vi "Form_motor_command.vi"(9 "Command selection":u16(ring)=1 items=["Move", "Get Motor Completed Steps (Q[0..3]C)", "Get Motor Direction (Q[0..3]D)", "Get Motor Step Rate: (Q[0..3]R)", "Get Switch State: (Q[0..3]S)"], 10 "Move parameters":T1={"MOTOR NUMBER"=0, "Direction"=TRUE, "NUMBER OF  STEPS"=8000, "SPEED STEPS/SEC"=2000, "ACC/DECEL STEPS/SEC^2"=1000, "Move mode"=1, "EN/DIS?"=TRUE, "delay before \nread (ms)"=750, "Timeout before \nstop (ms)"=15000, "visa resource name"=""} {"Move mode" items=["Relative steps ##", "Search switch"]; "ACC/DECEL STEPS/SEC^2" max=4000; "SPEED STEPS/SEC" min=20 max=4000 step=10; "MOTOR NUMBER" max=3 step=1}) -> (3 "Motor Command Formed":string)   [LabVIEW 2020]
panel:
  in  "Commands strings":string[](array[string])=["M01-R1000:100:1000\n", "Q0C", "Q0D", "Q0S", "Q0D"]
  # "Emergency Stop:\n *      [M]|Motor # [0-3]|Motor State [0]|[EOT]\n *\n *  Get Motor Completed Steps:\n *      [Q]|Motor # [0-3]|[C]|[EOT]\n *  Get Motor Direction:\n *      [Q]|Motor # [0-3]|[D]|[EOT]\n *  Get Motor Step Rate:\n *      [Q]|Motor # [0-3]|[R]|[EOT]\n *  Get Switch State:\n *      [Q]|Motor # [0-3]|[S]|[EOT]\n *\n *  Set Emergency Ramp Multiplier:\n *      [V]|Motor # [0-3]|[E]|Multiplier [uint]|[EOT]\n *\n *  Reset the arduino:\n *      [R]|[EOT]\n *"
  # "*  Move:\n *      [M]|Motor # [0-3]|Motor State [1]|Motor Direction [+,-]|Type of Move [R,S]|# Steps [uint]|Delimiter [:]|Max. Rate [uint]|Delimiter [:]|Ramp Slope [uint]|Delimiter [:] (optional)|# Positions [uint] (optional)|[EOT]\n *          * type of move: R --> relative move, S --> switch move\n *          * if number of steps is 0 --> free run\n *          * if Ramp Slope == 0 -> no ramp (start at max. rate)\n *          * may specify the number of position to move for a switch move.  if not specified, defaults to 1 position.\n *\n *  Emergency Stop:\n *      [M]|Motor # [0-3]|Motor State [0]|[EOT]\n *\n *  Get Motor Completed Steps:\n *      [Q]|Motor # [0-3]|[C]|[EOT]\n *  Get Motor Direction:\n *      [Q]|Motor # [0-3]|[D]|[EOT]\n *  Get Motor Step Rate:\n *      [Q]|Motor # [0-3]|[R]|[EOT]\n *  Get Switch State:\n *      [Q]|Motor # [0-3]|[S]|[EOT]\n *\n *  Set Emergency Ramp Multiplier:\n *      [V]|Motor # [0-3]|[E]|Multiplier [uint]|[EOT]\n */"
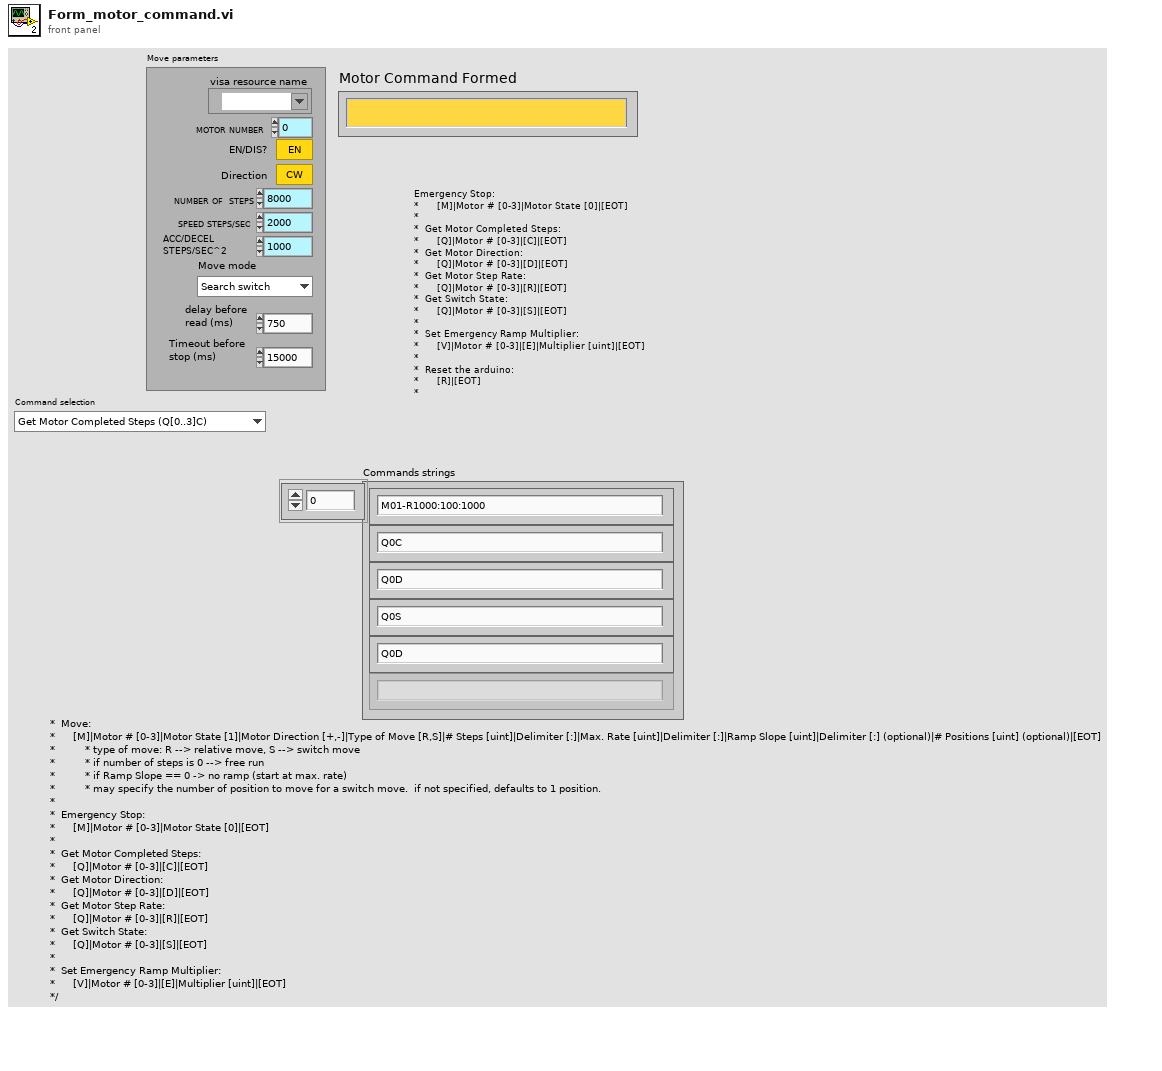
[diagram p1: front panel]
types:
  T1 = cluster{"MOTOR NUMBER":u8, "Direction":bool, "NUMBER OF  STEPS":u32, "SPEED STEPS/SEC":u16, "ACC/DECEL STEPS/SEC^2":u16, "Move mode":u16, "EN/DIS?":bool, "delay before \nread (ms)":u32, "Timeout before \nstop (ms)":u32, "visa resource name":refnum<visa-resource-name>}
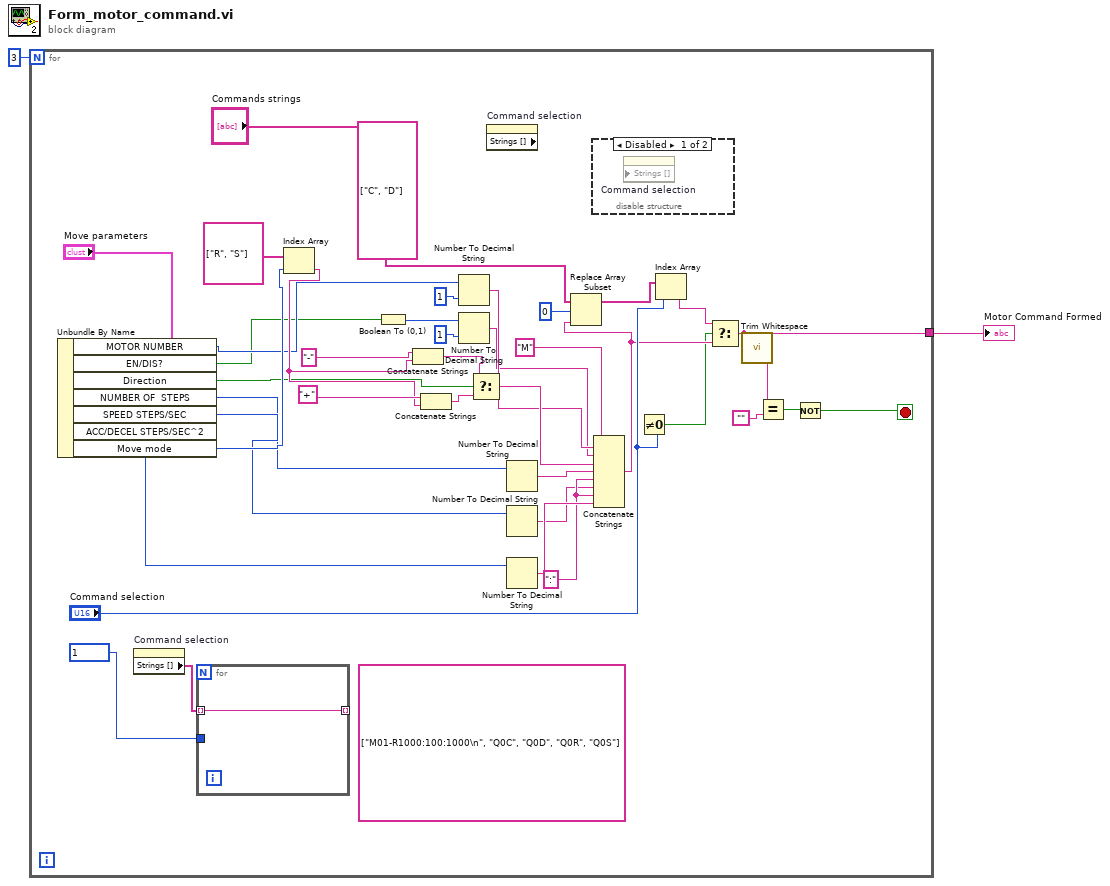
[diagram p0: block diagram]
diagram:
  n1 = for {
    N: 3 -> [_]
    tunnel: [w4] -> w1
    stop <- w5 stop-if-true
    (unwired) string[] ["M01-R1000:100:1000\n", "Q0C", "Q0D", "Q0R", "Q0S"] ("Commands strings")
    (unwired) string[] ["C", "D"]
    w22 = ":"
    n2 = Unbundle By Name("Move parameters") -> ("MOTOR NUMBER"=w14:u8, "EN/DIS?"=w12:bool, "Direction"=w30:bool, "NUMBER OF  STEPS"=w31:u32, "SPEED STEPS/SEC"=w32:u16, "ACC/DECEL STEPS/SEC^2"=w33:u16, "Move mode"=w41:u16)
    n3 = property on="Command selection" class="Ring (strict)"() -> ("Strings []"=w9:string[])  [unwired: 2 in, 2 out]
    n4 = for {
      tunnel: u16 1 ("Command selection") -> [_]
      tunnel: [w42] -> _ mode=indexing
      tunnel: w9 -> [w42] mode=indexing
    }
    n5 = Index Array(array=string[] ["R", "S"], index=w41) -> (element=w38:string)
    n6 = Boolean To (0,1)(Boolean=w12) -> (0, 1=w13:i16)
    n7 = Concatenate Strings("-", w38) -> (w35:string)
    n8 = Concatenate Strings("+", w38) -> (w40:string)
    n9 = Number To Decimal String(number=w14, width (-)=i16 1) -> (decimal integer string=w18:string)
    n10 = Number To Decimal String(number=w13, width (-)=i16 1) -> (decimal integer string=w11:string)
    n11 = Select(t=w35, s=w30, f=w40) -> (s? t:f=w27:string)
    n12 = property on="Command selection" class="Ring (strict)" props=["Strings []"]() -> ()  [unwired: 2 in, 3 out]
    n13 = Number To Decimal String(number=w31) -> (decimal integer string=w20:string)  [unwired: 1 in]
    n14 = Number To Decimal String(number=w32) -> (decimal integer string=w21:string)  [unwired: 1 in]
    n15 = Number To Decimal String(number=w33) -> (decimal integer string=w23:string)  [unwired: 1 in]
    n16 = disable-structure shown="Disabled" {
      frame Disabled {
        n17 = property on="Command selection" class="Ring (strict)" props=["Strings []"]() -> ()  [unwired: 3 in, 2 out]
      }
      frame Enabled {
      }
    }
    n18 = Concatenate Strings("M", w18, w11, w27, w20, w22, w21, w22, w23) -> (w28:string)
    n19 = Replace Array Subset(array="Commands strings", new element=w28, index=0) -> (w16:string[])
    n20 = Not Equal To 0?(x="Command selection") -> (x != 0?=w24:bool)
    n21 = Index Array(array=w16, index="Command selection") -> (element=w25:string)
    n22 = Select(t=w25, s=w24, f=w28) -> (s? t:f=w4:string)
    n23 = call <vilib>:"Trim Whitespace.vi"("string"=w4) -> ("trimmed string"=w3:string)  [unwired: 1 in]
    n24 = Equal?(x=w3, y="") -> (x = y?=w6:bool)
    n25 = Not(x=w6) -> (.not. x?=w5:bool)
  }
  "Motor Command Formed" <- w1
